vi "Configure Average.vi"(6 "Average Mode (1: Sweep)":i32(ring)=1 items=["Point", "Sweep"], 7 "Enable Average (F: Disable)":bool, 8 "error in (no error)":errorcluster, 9 "Average Count (1)":i32=1, 10 "Channel (1)":i32=1, 11 "VISA resource name":refnum<visa-resource-name>) -> (0 "error out":errorcluster, 3 "VISA resource name out":refnum<visa-resource-name>)   [LabVIEW 2018, in "Keysight PNA Series.lvlib"]
doc: "Configures sweep-to-sweep averaging parameters."
uses:
  Keysight PNA Series.lvlib
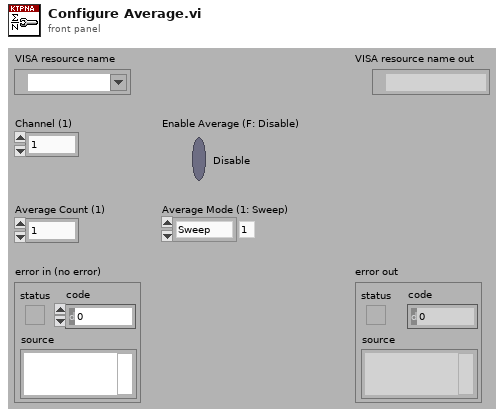
[diagram p1: front panel]
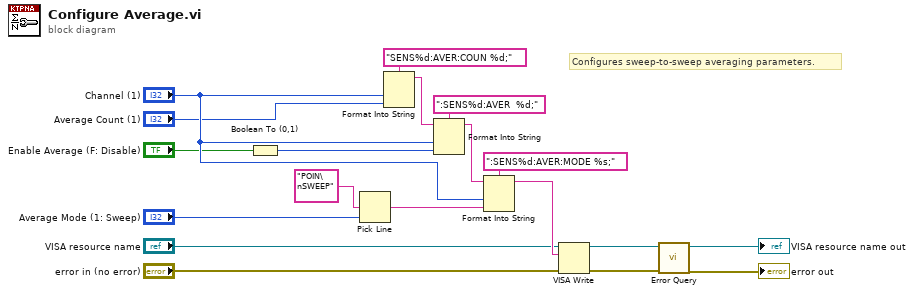
[diagram p0: block diagram]
diagram:
  # "Configures sweep-to-sweep averaging parameters."
  n1 = Boolean To (0,1)(Boolean="Enable Average (F: Disable)") -> (0, 1=w1:i16)
  n2 = Pick Line(multi-line string="POIN\nSWEEP", line index="Average Mode (1: Sweep)") -> (output string=w10:string)  [unwired: 1 in]
  n3 = Format Into String(format string="SENS%d:AVER:COUN %d;", "Channel (1)", "Average Count (1)") -> (resulting string=w16:string)  [unwired: 2 in, 1 out]
  n4 = Format Into String(format string=":SENS%d:AVER  %d;", initial string=w16, "Channel (1)", w1) -> (resulting string=w12:string)  [unwired: 1 in, 1 out]
  n5 = Format Into String(format string=":SENS%d:AVER:MODE %s;", initial string=w12, "Channel (1)", w10) -> (resulting string=w9:string)  [unwired: 1 in, 1 out]
  n6 = VISA Write(VISA resource name="VISA resource name", write buffer=w9, error in (no error)="error in (no error)") -> (VISA resource name out=w6:refnum<visa-resource-name>, error out=w5:errorcluster)  [unwired: 1 out]
  n7 = call "Error Query.vi"("error in (no error)"=w5, "VISA resource name"=w6) -> ("error out"=→"error out":errorcluster, "VISA resource name out"=→"VISA resource name out":refnum<visa-resource-name>)  [unwired: 6 in, 2 out]
